vi "message with stats c2s.vi"(0 "cluster":T1 {"message"."id" format="%x"; "message"."data" format="%x"}, 1 "add header? (F)":bool) -> (2 "string":string)   [LabVIEW 2024, in "atsj peakcan basic.lvlib"]
uses:
  atsj peakcan basic.lvlib
  message with stats.ctl
  message.ctl
  message type.ctl
  <vilib>/Utility/error.llb/Trim Whitespace.vi
  <vilib>/Utility/error.llb/Trim Whitespace One-Sided.vi
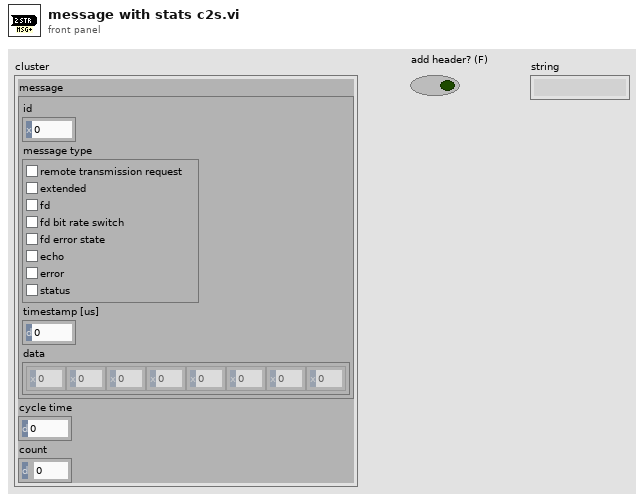
[diagram p1: front panel]
types:
  T1 = typedef "atsj peakcan basic.lvlib/message with stats.ctl" = cluster{"message":T2, "cycle time":u64, "count":u64}
  T2 = typedef "atsj peakcan basic.lvlib/message.ctl" = cluster{"id":u32, "message type":T3, "timestamp [us]":u64, "data":u8[]}
  T3 = typedef "atsj peakcan basic.lvlib/message type.ctl" = cluster{"remote transmission request ":bool, "extended":bool, "fd":bool, "fd bit rate switch":bool, "fd error state":bool, "echo":bool, "error":bool, "status":bool}
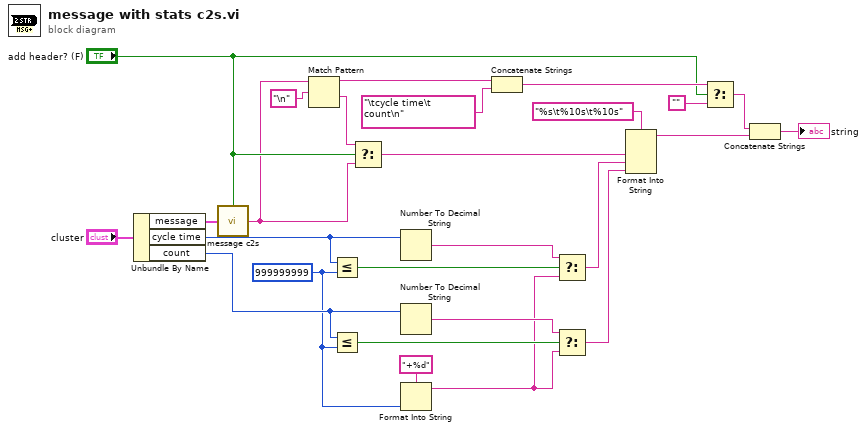
[diagram p0: block diagram]
diagram:
  w12 = u64 999999999
  n1 = Unbundle By Name("cluster") -> ("message"=w9:T2, "cycle time"=w20:u64, "count"=w19:u64)
  n2 = call "message c2s.vi"("cluster"=w9, "add header? (F)"="add header? (F)") -> ("string"=w2:string)
  n3 = Match Pattern(string=w2, regular expression="\n") -> (before substring=w7:string, after substring=w3:string)  [unwired: 1 in, 2 out]
  n4 = Less Or Equal?(x=w20, y=w12) -> (x <= y?=w18:bool)
  n5 = Less Or Equal?(x=w19, y=w12) -> (x <= y?=w15:bool)
  n6 = Select(t=w3, s="add header? (F)", f=w2) -> (s? t:f=w1:string)
  n7 = Number To Decimal String(number=w20) -> (decimal integer string=w17:string)  [unwired: 1 in]
  n8 = Number To Decimal String(number=w19) -> (decimal integer string=w16:string)  [unwired: 1 in]
  n9 = Format Into String(format string="+%d", w12) -> (resulting string=w11:string)  [unwired: 2 in, 1 out]
  n10 = Concatenate Strings(w7, "\tcycle time\t     count\n") -> (w5:string)
  n11 = Select(t=w17, s=w18, f=w11) -> (s? t:f=w14:string)
  n12 = Select(t=w16, s=w15, f=w11) -> (s? t:f=w13:string)
  n13 = Format Into String(format string="%s\t%10s\t%10s", w1, w14, w13) -> (resulting string=w23:string)  [unwired: 2 in, 1 out]
  n14 = Select(t=w5, s="add header? (F)", f="") -> (s? t:f=w24:string)
  n15 = Concatenate Strings(w24, w23) -> (→"string":string)
